vi "RefPosition.vi"(0 "X":dbl, 1 "Y":dbl, 2 "Z":dbl) -> ()   [LabVIEW 2017]
uses:
  Settings/Traverse-Settings-Global.vi
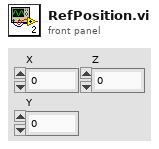
[diagram p1: front panel]
types:
  T1 = typedef "Settings-Control.ctl" = cluster{"Acceleration":dbl[], "Deceleration":dbl[], "Max Velocity":dbl[], "Speed":dbl, "Pulse/Degree":dbl, "Degre Factor":dbl[], "mm/rotation":dbl[], "Traverse Name":string}
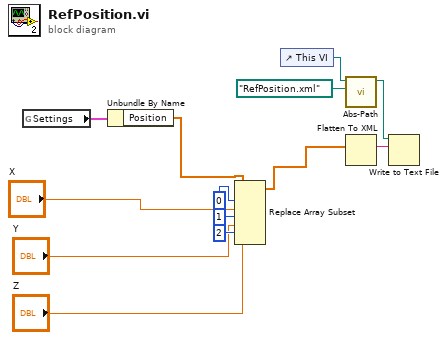
[diagram p0: block diagram]
diagram:
  n1 = global read "Traverse-Settings-Global.vi" "Settings"() -> (w9:T1)
  n2 = Unbundle By Name(w9) -> ("Position"=w5:dbl[])
  n3 = Replace Array Subset(array=w5, new element #1="X", index #1=0 ("index"), new element #2="Y", index #2=1 ("index"), new element #3="Z", index #3=2 ("index")) -> (w4:dbl[])
  n4 = control-ref of="This VI"() -> (w12:refnum<vi>)
  n5 = call "Abs-Path.vi"("filename"=path "RefPosition.xml" ("file (use dialog)"), "Vi in path"=w12) -> ("Full path"=w13:path)  [unwired: 9 in]
  n6 = Flatten To XML(anything=w4) -> (xml string=w11:string)
  n7 = Write to Text File(file (use dialog)=w13, text=w11) -> ()  [unwired: 2 in, 3 out]
